vi "PM_Synch_Monitor.vi"(7 "Polling Interval":u32=125, 8 "error in":errorcluster, 10 "Status In":T1, 11 "Synch In":refnum<k15>) -> (0 "error out":errorcluster, 1 "Synchronized?":bool, 2 "Status Out":T1, 3 "Reference out":refnum<k15>, 5 "Offset from TR (ns)":dbl)   [LabVIEW 2021]
uses:
  TypeDef/Synch_shift--cluster.ctl
panel:
  out "Selected TR Name":string
  out "Current Sync Duration (ms)":u32
  out "Sync Loss Count":u32
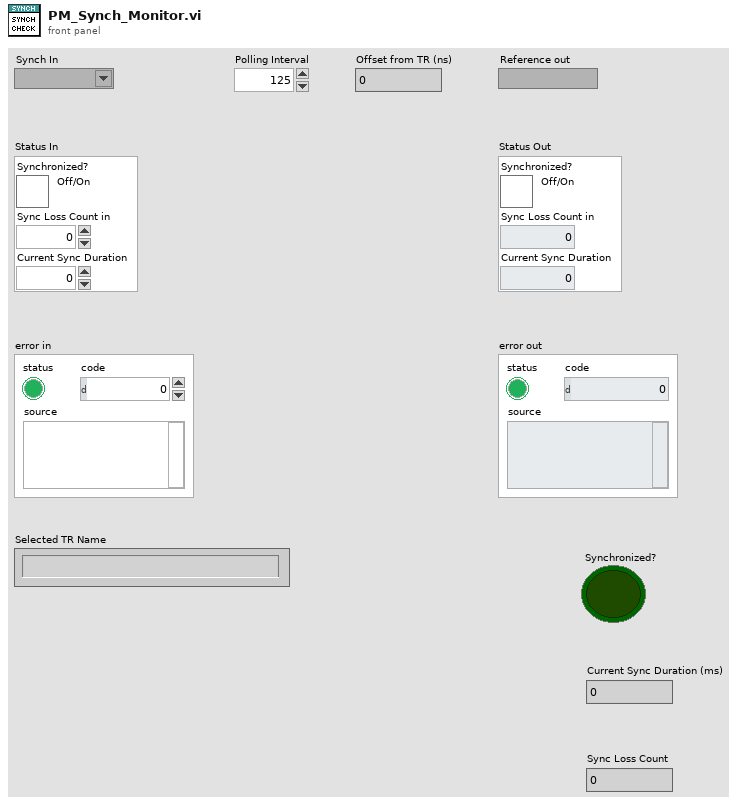
[diagram p1: front panel]
types:
  T1 = typedef "Synch_shift--cluster.ctl" = cluster{"Synchronized?":bool, "Sync Loss Count in":u32, "Current Sync Duration":u32}
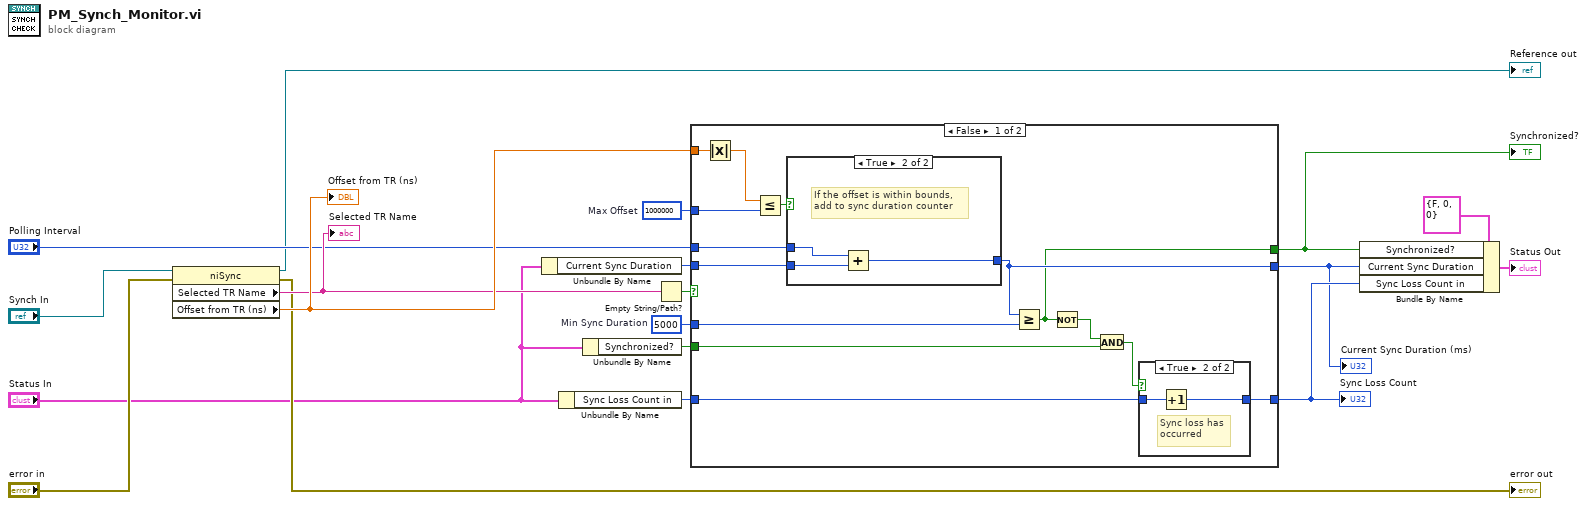
[diagram p0: block diagram]
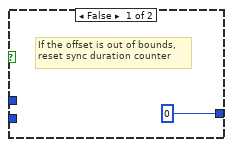
[diagram p3: hidden frame]
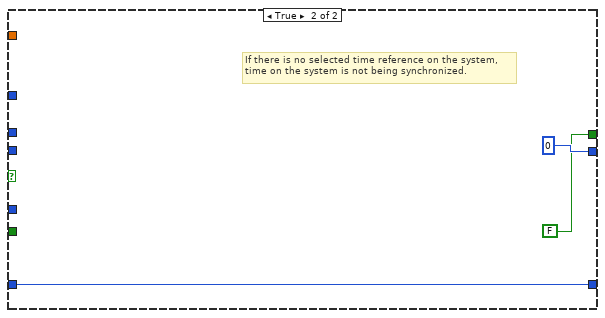
[diagram p4: hidden frame]
diagram:
  w15 = u32 5000  # Min Sync Duration
  w14 = 1000000  # Max Offset
  n1 = property class="niSync"(reference="Synch In", error in="error in") -> (reference out=→"Reference out":refnum<k15>, error out=→"error out":errorcluster, "Selected TR Name"=w17:string, "Offset from TR (ns)"=w19:dbl)
  "Selected TR Name" <- w17
  "Offset from TR (ns)" <- w19
  n2 = Unbundle By Name("Status In") -> ("Current Sync Duration"=w6:u32)
  n3 = Unbundle By Name("Status In") -> ("Sync Loss Count in"=w4:u32)
  n4 = Unbundle By Name("Status In") -> ("Synchronized?"=w5:bool)
  n5 = Empty String/Path?(string/path=w17) -> (empty?=w18:bool)
  n6 = case shown="False" w18 {
    tunnel: w5 -> [w32 _]
    tunnel: w4 -> [w29 w42]
    tunnel: w19 -> [w28 _]
    tunnel: w14 -> [w26 _]
    tunnel: [w21 u32 0] -> w1
    tunnel: [w20 FALSE] -> w8
    tunnel: w6 -> [w25 _]
    tunnel: "Polling Interval" -> [w24 _]
    tunnel: [w23 w42] -> w2
    tunnel: w15 -> [w22 _]
    frame False {
      n7 = Absolute Value(x=w28) -> (abs(x)=w27:dbl)
      n8 = Less Or Equal?(x=w27, y=w26) -> (x <= y?=w33:bool)
      n9 = case shown="True" w33 {
        tunnel: [u32 0 w40] -> w21
        tunnel: w24 -> [_ w39]
        tunnel: w25 -> [_ w38]
        frame False {
          # "If the offset is out of bounds,\nreset sync duration counter"
        }
        frame True {
          # "If the offset is within bounds,\nadd to sync duration counter"
          n10 = Add(x=w39, y=w38) -> (x+y=w40:u32)
        }
      }
      n11 = Greater Or Equal?(x=w21, y=w22) -> (x >= y?=w20:bool)
      n12 = Not(x=w20) -> (.not. x?=w31:bool)
      n13 = And(x=w31, y=w32) -> (x .and. y?=w30:bool)
      n14 = case shown="True" w30 {
        tunnel: w29 -> [w34 w36]
        tunnel: [w34 w35] -> w23
        frame False {
        }
        frame True {
          # "Sync loss has\noccurred"
          n15 = Increment(x=w36) -> (x+1=w35:u32)
        }
      }
    }
    frame True {
      # "If there is no selected time reference on the system,\ntime on the system is not being synchronized."
    }
  }
  "Current Sync Duration (ms)" <- w1
  "Sync Loss Count" <- w2
  "Synchronized?" <- w8
  n16 = Bundle By Name(cluster=T1 {"Synchronized?"=FALSE, "Sync Loss Count in"=0, "Current Sync Duration"=0} ("Status Out"), "Synchronized?"=w8, "Current Sync Duration"=w1, "Sync Loss Count in"=w2) -> (→"Status Out":T1)
